vi "solar_cfg Write File (Var).vi"(0 "Config Path (*.ini)":path, 1 "Section (\"\" = Use Filename)":string, 2 "Comments (Key,Comment)":cluster{"Key":string, "Comment":string}[](array[cluster]), 5 "Key_Prefix (\"\")":string, 7 "Variant":variant, 11 "error in (no error)":errorcluster, 12 "ArrayDelimiters (1D,2D)":string[](array[string])) -> (4 "Config Path out":path, 10 "Found?":bool, 15 "error out":errorcluster)   [LabVIEW 2018]
doc: "Write the values associated with a variant to a specified section in the configuration file. If the Key is empty the variant label is used instead. Set a Comment (#...) to add a description after the key's value. Clusters use the element lables are their key names. Set Enum as Strings to True to use the string item of an enum.\n\nSupported Data Types: \nI8..EXT, Enum, Boolean, String, Path, VISA Reference, Timestamp\n1D & 2D Arrays and Clusters of the data types above.\n\n[Section]\nKey = \"Value\" #Comment"
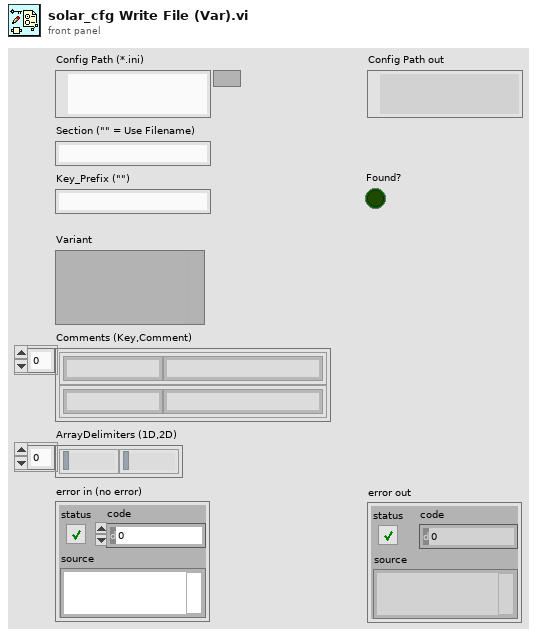
[diagram p1: front panel]
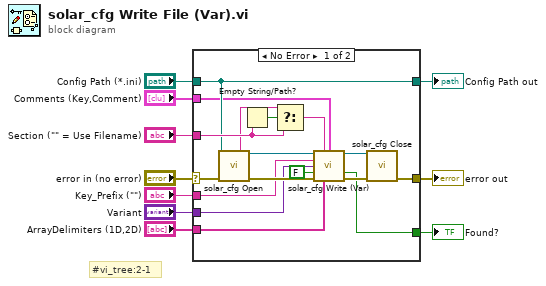
[diagram p0: block diagram]
diagram:
  # "#vi_tree:2-1"
  n1 = case shown="No Error" "error in (no error)" {
    selector: "error in (no error)" -> [w25 w29]
    tunnel: "Config Path (*.ini)" -> [w24 w28]
    tunnel: [w22 w29] -> w8
    tunnel: "Section (\"\" = Use Filename)" -> [w26 _]
    tunnel: [w24 w28] -> w6
    tunnel: "Variant" -> [w14 _]
    tunnel: [w12 _] -> w4
    tunnel: "Key_Prefix (\"\")" -> [w15 _]
    tunnel: "Comments (Key,Comment)" -> [w16 _]
    tunnel: "ArrayDelimiters (1D,2D)" -> [w13 _]
    frame No Error {
      n2 = call "solar_cfg Open.vi"("Config Path (*.ini)"=w24, "error in (no error)"=w25) -> ("Filename"=w23:string, "Config Refnum"=w21:refnum<data-value>, "error out"=w20:errorcluster)  [unwired: 10 in, 1 out]
      n3 = Empty String/Path?(string/path=w26) -> (empty?=w27:bool)
      n4 = Select(t=w23, s=w27, f=w26) -> (s? t:f=w17:string)
      n5 = call "solar_cfg Write (Var).vi"("Config Refnum"=w21, "Section"=w17, "Comments (Key,Comment)"=w16, "Key (\"\")"=w15, "Variant"=w14, "Include Variant Name? (F)"=FALSE ("Include Cluster Name? (F)"), "error in (no error)"=w20, "ArrayDelimiters (1D,2D)"=w13) -> ("dup Config Refnum"=w18:refnum<data-value>, "Found?"=w12:bool, "error out"=w19:errorcluster)  [unwired: 5 in]
      n6 = call "solar_cfg Close.vi"("Config Refnum"=w18, "error in (no error)"=w19) -> ("error out"=w22:errorcluster)  [unwired: 12 in, 1 out]
    }
    frame Error {
    }
  }
  "error out" <- w8
  "Config Path out" <- w6
  "Found?" <- w4
